vi "ObtenerDatosdelatabla.vi"(9 "Column":i32, 10 "Row":i32, 11 "Prueba32 in":refnum<class "Prueba32.lvclass">) -> (3 "Prueba32 out":refnum<class "Prueba32.lvclass">)   [LabVIEW 2019, in "Prueba32.lvclass"]
uses:
  Prueba32.lvclass
  Prueba32.lvclass/Prueba32.ctl
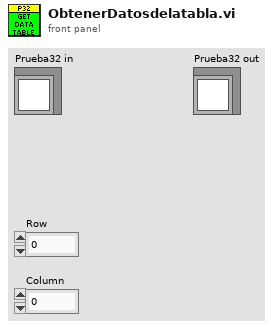
[diagram p1: front panel]
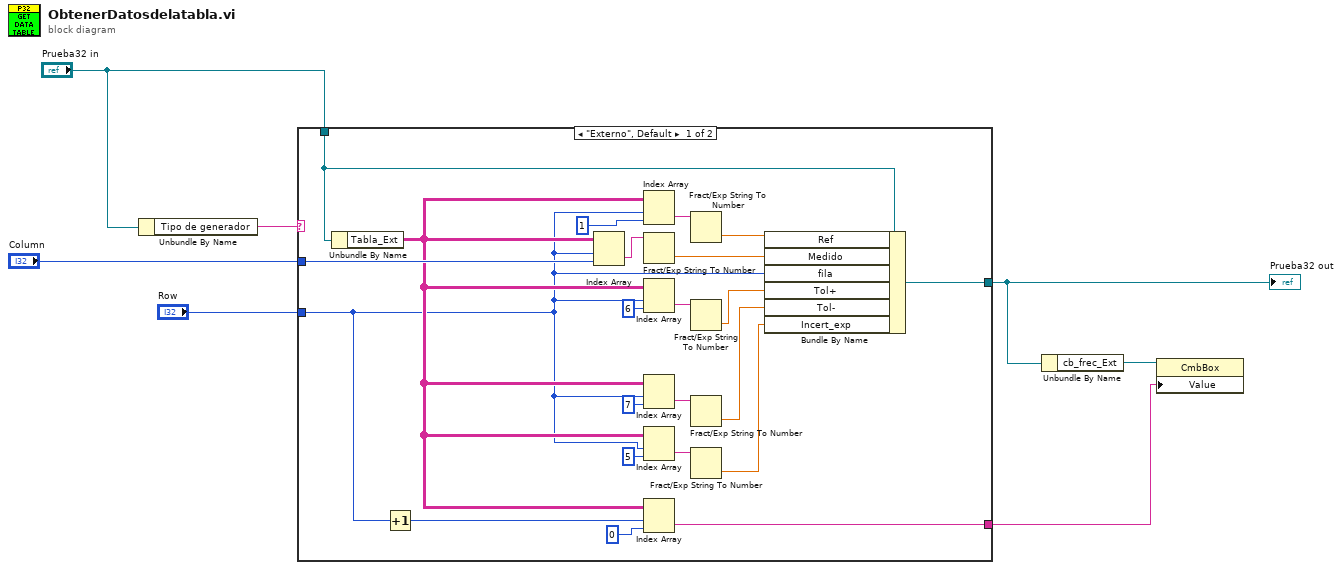
[diagram p0: block diagram]
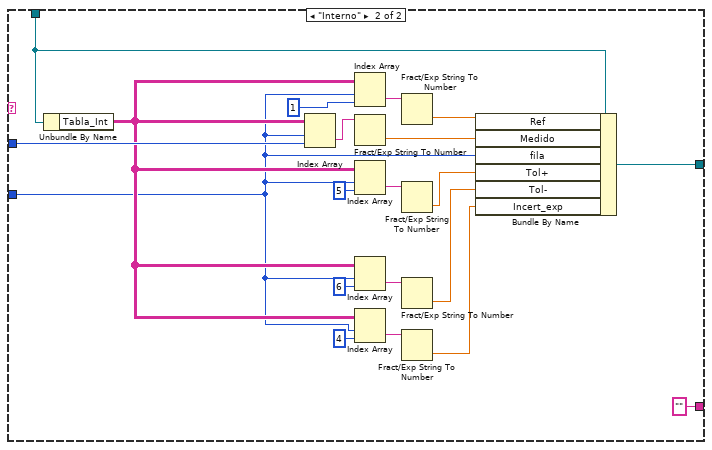
[diagram p2: hidden frame]
diagram:
  n1 = Unbundle By Name("Prueba32 in") -> ("Tipo de generador"=w4:string)
  n2 = case shown="\"Externo\", Default" w4 {
    tunnel: "Row" -> [w11 w31]
    tunnel: [w15 w35] -> w3
    tunnel: "Column" -> [w14 w34]
    tunnel: "Prueba32 in" -> [w13 w33]
    tunnel: [w9 "" ("tipo dato")] -> w1
    frame "Externo", Default {
      n3 = Unbundle By Name(w13) -> ("Tabla_Ext"=w12:string[][])
      n4 = Increment(x=w11) -> (x+1=w8:i32)
      n5 = Index Array(array=w12, index (row)=w11, index (col)=w14) -> (element=w16:string)
      n6 = Index Array(array=w12, index (row)=w11, index (col)=1 ("disabled index (col)")) -> (element=w19:string)
      n7 = Fract/Exp String To Number(string=w16) -> (number=w17:dbl)  [unwired: 3 in, 1 out]
      n8 = Index Array(array=w12, index (row)=w11, index (col)=6 ("disabled index (col)")) -> (element=w21:string)
      n9 = Index Array(array=w12, index (row)=w11, index (col)=7 ("disabled index (col)")) -> (element=w24:string)
      n10 = Index Array(array=w12, index (row)=w11, index (col)=5 ("disabled index (col)")) -> (element=w28:string)
      n11 = Index Array(array=w12, index (row)=w8, index (col)=0 ("disabled index (col)")) -> (element=w9:string)
      n12 = Fract/Exp String To Number(string=w19) -> (number=w20:dbl)  [unwired: 3 in, 1 out]
      n13 = Fract/Exp String To Number(string=w21) -> (number=w22:dbl)  [unwired: 3 in, 1 out]
      n14 = Fract/Exp String To Number(string=w24) -> (number=w25:dbl)  [unwired: 3 in, 1 out]
      n15 = Fract/Exp String To Number(string=w28) -> (number=w29:dbl)  [unwired: 3 in, 1 out]
      n16 = Bundle By Name(cluster=w13, "Ref"=w20, "Medido"=w17, "fila"=w11, "Tol+"=w22, "Tol-"=w25, "Incert_exp"=w29) -> (w15:refnum<class "Prueba32.lvclass">)
    }
    frame "Interno" {
      n17 = Unbundle By Name(w33) -> ("Tabla_Int"=w32:string[][])
      n18 = Index Array(array=w32, index (row)=w31, index (col)=w34) -> (element=w36:string)
      n19 = Index Array(array=w32, index (row)=w31, index (col)=1 ("disabled index (col)")) -> (element=w39:string)
      n20 = Fract/Exp String To Number(string=w36) -> (number=w37:dbl)  [unwired: 3 in, 1 out]
      n21 = Index Array(array=w32, index (row)=w31, index (col)=5 ("disabled index (col)")) -> (element=w41:string)
      n22 = Index Array(array=w32, index (row)=w31, index (col)=6 ("disabled index (col)")) -> (element=w44:string)
      n23 = Index Array(array=w32, index (row)=w31, index (col)=4 ("disabled index (col)")) -> (element=w48:string)
      n24 = Fract/Exp String To Number(string=w39) -> (number=w40:dbl)  [unwired: 3 in, 1 out]
      n25 = Fract/Exp String To Number(string=w41) -> (number=w42:dbl)  [unwired: 3 in, 1 out]
      n26 = Fract/Exp String To Number(string=w44) -> (number=w45:dbl)  [unwired: 3 in, 1 out]
      n27 = Fract/Exp String To Number(string=w48) -> (number=w49:dbl)  [unwired: 3 in, 1 out]
      n28 = Bundle By Name(cluster=w33, "Ref"=w40, "Medido"=w37, "fila"=w31, "Tol+"=w42, "Tol-"=w45, "Incert_exp"=w49) -> (w35:refnum<class "Prueba32.lvclass">)
    }
  }
  "Prueba32 out" <- w3
  n29 = Unbundle By Name(w3) -> ("cb_frec_Ext"=w2:refnum<vi>)
  n30 = property class="CmbBox"(reference=w2, "Value"=w1) -> ()  [unwired: 1 in, 2 out]
